vi "电阻采集.vi"(8 "error in (no error)":errorcluster, 11 "Keithley2750":refnum<visa-resource-name>="GPIB0::16::INSTR") -> (0 "error out":errorcluster caption="错误输出", 2 "多通道温度值":dbl[](array[numeric]))   [LabVIEW 2015]
uses:
  Keithley 27XX/Keithley 27XX.lvlib
  <vilib>/Analysis/NI_AALBase.lvlib
  <vilib>/Analysis/baseanly.llb/Mean (DBL).vi
panel:
  out "VISA引用句柄输出":refnum<visa-resource-name>
  out "测量结果":dbl
  out "Scan List (Empty: front panel)":string
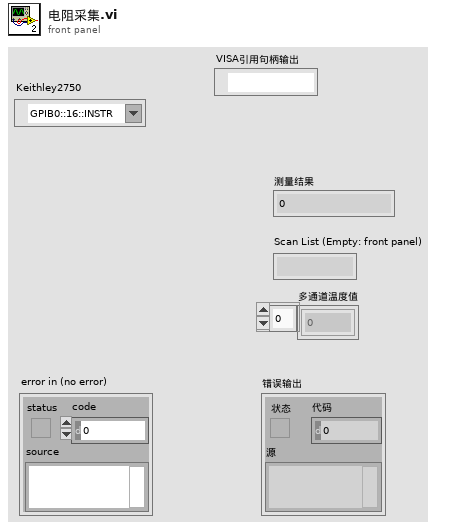
[diagram p1: front panel]
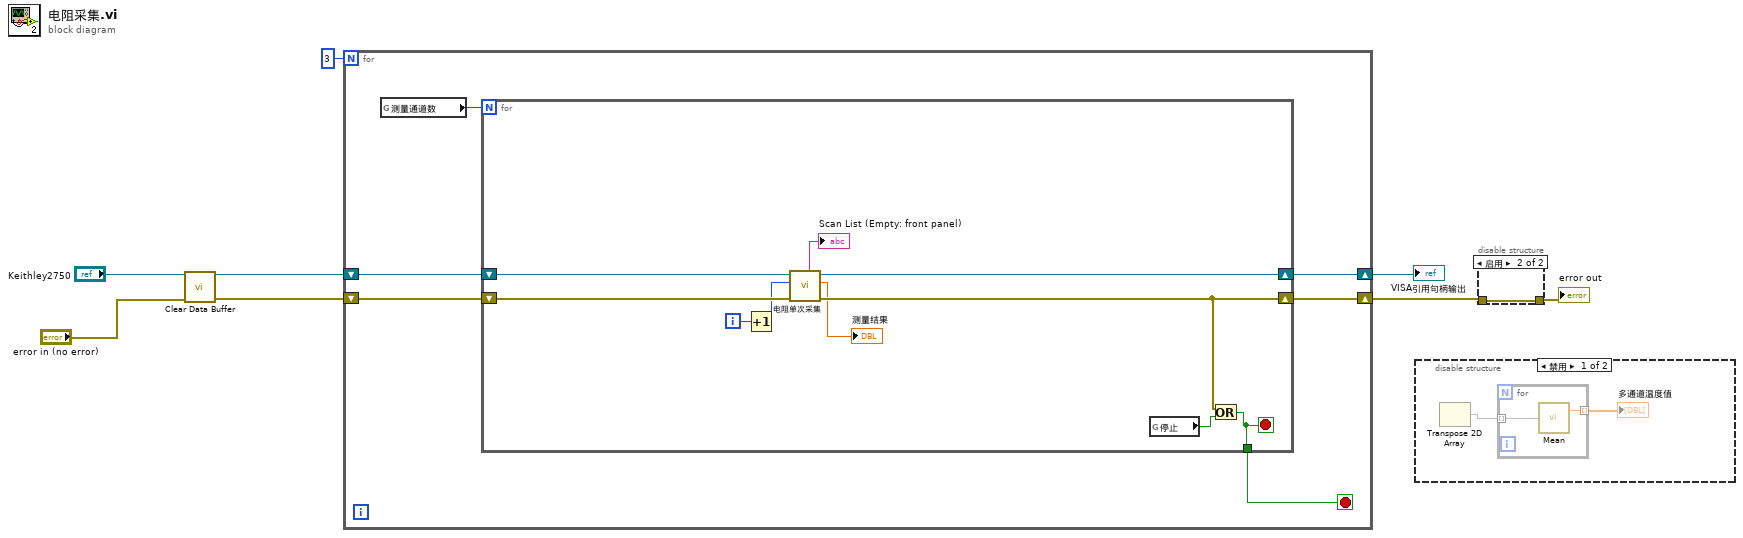
[diagram p0: block diagram]
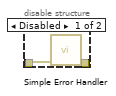
[diagram p3: hidden frame]
diagram:
  n1 = call "Clear Data Buffer.vi"("VISA resource name"="Keithley2750", "error in (no error)"="error in (no error)") -> ("VISA resource name out"=w7:refnum<visa-resource-name>, "error out"=w8:errorcluster)  [unwired: 12 in]
  n2 = for {
    N: 3 -> [_]
    shift-right: [w13] -> w2
    shift-left: w8 -> [w12]
    shift-right: [w14] -> w1
    shift-left: w7 -> [w11]
    stop <- w10 stop-if-true
    n3 = global read "全局.vi" "测量通道数"() -> (w9:i32)
    n4 = for {
      N: w9 -> [_]
      shift-right: [w21] -> w13
      shift-left: w12 -> [w24]
      shift-right: [w22] -> w14
      shift-left: w11 -> [w23]
      tunnel: [w19] -> w10
      i -> [w17]
      stop <- w19 stop-if-true
      n5 = Increment(x=w17) -> (x+1=w16:i32)
      n6 = call "电阻单次采集.vi"("错误输入（无错误）"=w24, "通道数"=w16, "VISA引用句柄输入"=w23) -> ("错误输出"=w21:errorcluster, "测量结果"=→"测量结果":dbl, "VISA引用句柄输出"=w22:refnum<visa-resource-name>, "Scan List (Empty: front panel)"=→"Scan List (Empty: front panel)":string)  [unwired: 5 in]
      n7 = global read "全局.vi" "停止"() -> (w20:bool)
      n8 = Or(x=w21, y=w20) -> (x .or. y?=w19:bool)
    }
  }
  "VISA引用句柄输出" <- w1
  n9 = disable-structure shown="禁用" {
    frame Disabled {
      n10 = Transpose 2D Array() -> (transposed array=w26:dbl[][])  [unwired: 1 in]
      n11 = for {
        tunnel: w26 -> [w28] mode=indexing
        tunnel: [w27] -> w25 mode=indexing
        n12 = call-poly <vilib>:"Mean.vi"("X"=w28) -> ("mean"=w27:dbl)  [unwired: 1 out]
      }
      "多通道温度值" <- w25
    }
    frame Enabled {
    }
  }
  n13 = disable-structure shown="启用" {
    disable-tunnel: [w30 w31] -> w5
    disable-tunnel: w2 -> [w29 w31]
    frame Disabled {
      n14 = call <vilib>:"Simple Error Handler.vi"("error in (no error)"=w29) -> ("error out"=w30:errorcluster)  [unwired: 4 in, 4 out]
    }
    frame Enabled {
    }
  }
  "error out" <- w5
